vi "ReadAndPreprocessSensorValues.vi"(6 "Sensor References":T12, 8 "Force_calib_value":dbl, 9 "Velocity_calib_value":dbl, 10 "Control Loop Period [s]":dbl, 11 "Time [s]":dbl) -> (3 "RobotStateType":T13)   [LabVIEW 2019]
uses:
  ClusterType/RobotStateType.ctl
  <vilib>/myRIO/Instrument Drivers/Onboard IO/Encoder/typedefs/Encoder Reference.ctl
  <vilib>/myRIO/Common/Instrument Driver Framework/Utilities/typedefs/myRIO Generic Hardware Reference.ctl
  <vilib>/myRIO/Common/Instrument Driver Framework/Utilities/typedefs/Hardware Version Enum.ctl
  <vilib>/myRIO/Common/Instrument Driver Framework/Utilities/typedefs/myRIO v1.0 Reference.ctl
  <vilib>/myRIO/Common/Instrument Driver Framework/Utilities/typedefs/Generic FPGA Reference.ctl
  <vilib>/myRIO/Common/Instrument Driver Framework/myRIO v1.0/Encoder/typedefs/Encoder Channels Enum.ctl
  <vilib>/myRIO/Instrument Drivers/Onboard IO/AI/typedefs/AI Reference.ctl
  <vilib>/myRIO/Common/Instrument Driver Framework/myRIO v1.0/AI/typedefs/AI Channels List.ctl
  <vilib>/myRIO/Common/Instrument Driver Framework/myRIO v1.0/AI/typedefs/AI Channels Enum.ctl
  <vilib>/myRIO/Common/Instrument Driver Framework/Utilities/typedefs/Analog Scaling Constants List.ctl
  <vilib>/myRIO/Common/Instrument Driver Framework/Utilities/typedefs/Analog Scaling Constants.ctl
  <vilib>/Analysis/3filter.llb/Filter Passband Type.ctl
  <vilib>/Utility/error.llb/Error Cluster From Error Code.vi
  <vilib>/myRIO/Common/Instrument Driver Framework/myRIO v1.0/AI/vis/myRIO v1.0 Read AI.vi
  <vilib>/myRIO/Common/Instrument Driver Framework/myRIO v1.0/Encoder/vis/myRIO v1.0 Read Encoder.vi
  <vilib>/myRIO/Instrument Drivers/Onboard IO/Encoder/Encoder.lvlib
  <vilib>/myRIO/Instrument Drivers/Onboard IO/AI/AI.lvlib
  <vilib>/Analysis/NI_AALBase.lvlib
  <vilib>/ptbypt/NI_PtbyPt.lvlib
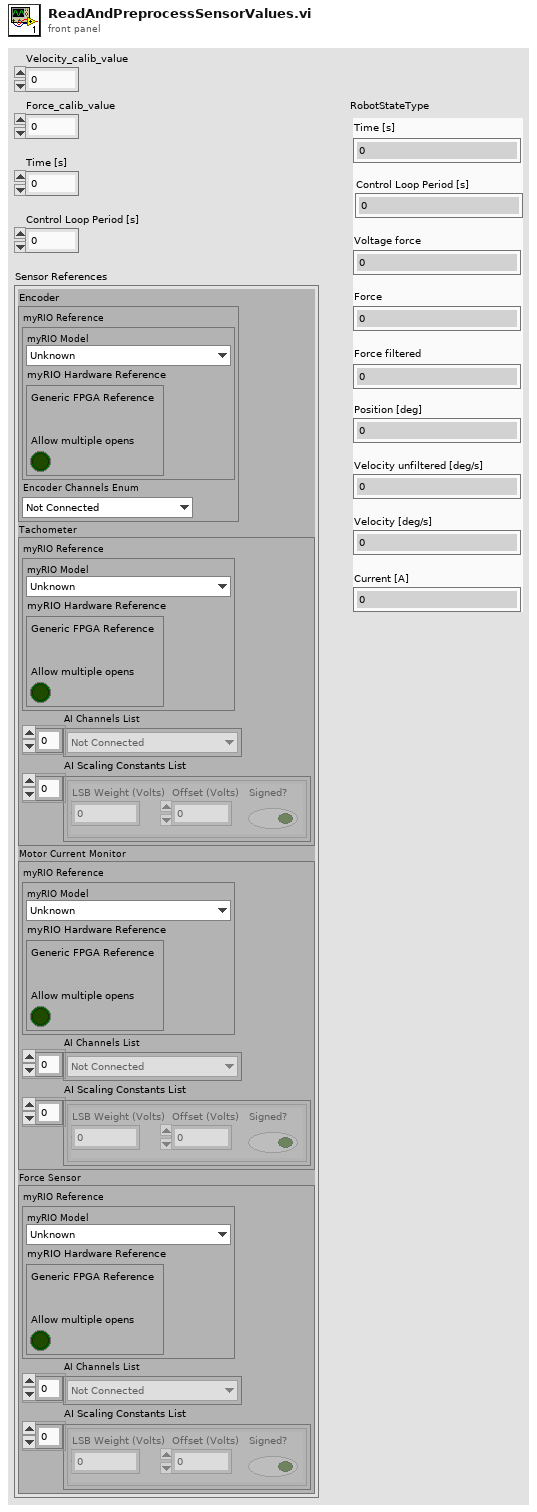
[diagram p1: front panel]
types:
  T1 = typedef "Encoder.lvlib/Encoder Reference.ctl" = cluster{"myRIO Reference":T2, "Encoder Channels Enum":T6}
  T2 = typedef "myRIO Generic Hardware Reference.ctl" = cluster{"myRIO Model":T3, "myRIO Hardware Reference":T4}
  T3 = typedef "Hardware Version Enum.ctl" = enum16{"Unknown", "myRIO-1900", "myRIO-1950", "roboRIO", "NI ELVIS RIO CM", "ELVIS III"}
  T4 = typedef "myRIO v1.0 Reference.ctl" = cluster{"Generic FPGA Reference":T5, "Allow multiple opens":bool}
  T5 = typedef "Generic FPGA Reference.ctl" = refnum<k20>
  T6 = typedef "Encoder Channels Enum.ctl" = enum16{"Not Connected", "C/ENC0", "C/ENC1", "A/ENC", "A/ENC0", "A/ENC1", "A/ENC2", "A/ENC3", "A/ENC4", "A/ENC5", "A/ENC6", "A/ENC7", "A/ENC8", "A/ENC9", "B/ENC", "B/ENC0", "B/ENC1", "B/ENC2", "B/ENC3", "B/ENC4", "B/ENC5", "B/ENC6", "B/ENC7", "B/ENC8", "B/ENC9", "DIO/ENC0", "DIO/ENC1", "DIO/ENC2", "DIO/ENC3", "DIO/ENC4"}
  T7 = typedef "AI.lvlib/AI Reference.ctl" = cluster{"myRIO Reference":T2, "AI Channels List":T8, "AI Scaling Constants List":T10}
  T8 = typedef "AI Channels List.ctl" = T9[]
  T9 = typedef "AI Channels Enum.ctl" = enum16{"Not Connected", "AudioIn/Left", "AudioIn/Right", "C/AI0", "C/AI1", "A/AI0", "A/AI1", "A/AI2", "A/AI3", "A/AI4", "A/AI5", "A/AI6", "A/AI7", "B/AI0", "B/AI1", "B/AI2", "B/AI3", "B/AI4", "B/AI5", "B/AI6", "B/AI7", "AI/AI0", "AI/AI1", "AI/AI2", "AI/AI3", "A/AI0 (DIFF)", "A/AI1 (DIFF)", "A/AI2 (DIFF)", "A/AI3 (DIFF)", "B/AI0 (DIFF)", "B/AI1 (DIFF)", "B/AI2 (DIFF)", "B/AI3 (DIFF)"}
  T10 = typedef "Analog Scaling Constants List.ctl" = T11[]
  T11 = typedef "Analog Scaling Constants.ctl" = cluster{"LSB Weight (Volts)":dbl, "Offset (Volts)":dbl, "Signed?":bool}
  T12 = cluster{"Encoder":T1, "Tachometer":T7, "Motor Current Monitor":T7, "Force Sensor":T7}
  T13 = typedef "RobotStateType.ctl" = cluster{"Time [s]":dbl, "Voltage force":dbl, "Force":dbl, "Force filtered":dbl, "Position [deg]":dbl, "Velocity unfiltered [deg/s]":dbl, "Velocity [deg/s]":dbl, "Current [A]":dbl, "Control Loop Period [s]":dbl}
  T14 = typedef "NI_AALBase.lvlib/Filter Passband Type.ctl" = enum32{"Lowpass", "Highpass", "Bandpass", "Bandstop"}
  T15 = typedef "TypeDefTachometerParam.ctl" = cluster{"Offset [V]":dbl, "Gain [deg/sV]":dbl}
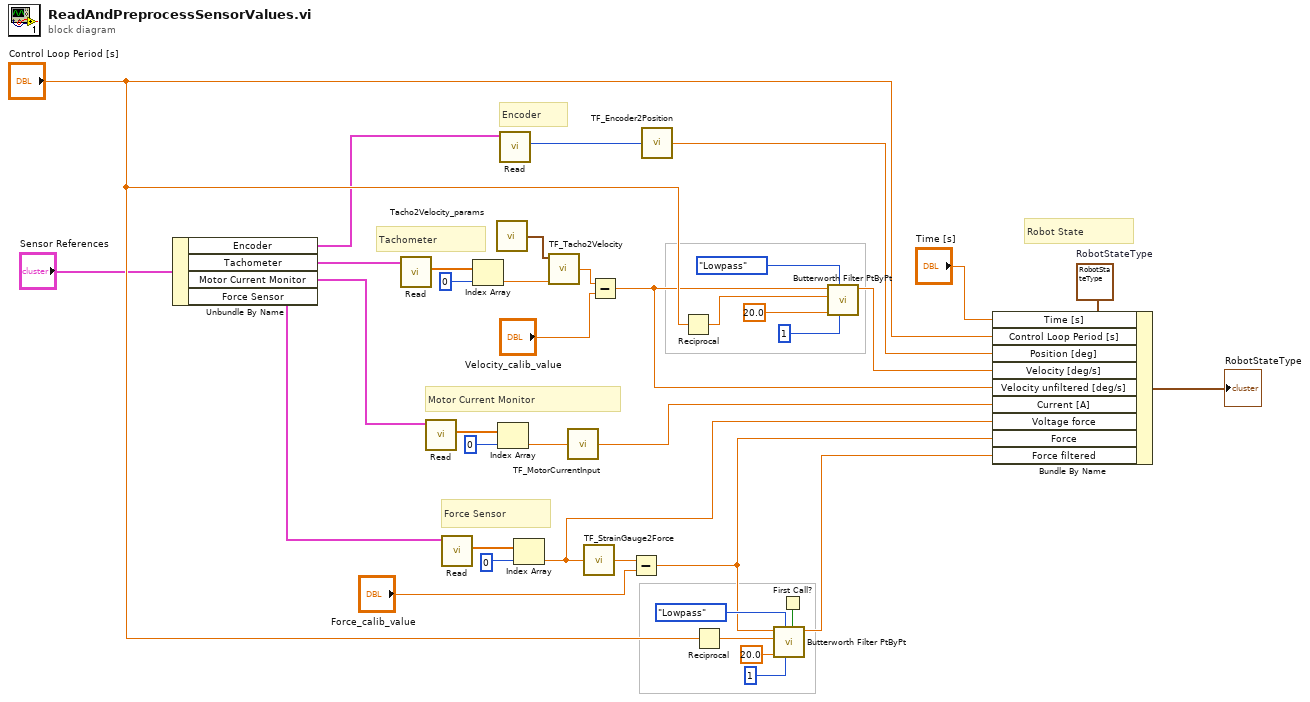
[diagram p0: block diagram]
diagram:
  w32 = T13 {"Time [s]"=0.0, "Voltage force"=0.0, "Force"=0.0, "Force filtered"=0.0, "Position [deg]"=0.0, "Velocity unfiltered [deg/s]"=0.0, "Velocity [deg/s]"=0.0, "Current [A]"=0.0, "Control Loop Period [s]"=0.0}  # RobotStateType
  # "Robot State"
  # "Force Sensor"
  # "Motor Current Monitor"
  # "Tachometer"
  # "Encoder"
  n1 = Unbundle By Name("Sensor References") -> ("Encoder"=w28:T1, "Tachometer"=w29:T7, "Motor Current Monitor"=w30:T7, "Force Sensor"=w31:T7)
  n2 = call <vilib>:"Read.vi"("AI Ref In"=w29) -> ("Values"=w10:dbl[])  [unwired: 8 in, 2 out]
  n3 = call <vilib>:"Read.vi"("AI Ref In"=w30) -> ("Values"=w11:dbl[])  [unwired: 8 in, 2 out]
  n4 = call <vilib>:"Read.vi"("AI Ref In"=w31) -> ("Values"=w15:dbl[])  [unwired: 8 in, 2 out]
  n5 = Index Array(array=w10, index=0) -> (element=w6:dbl)
  n6 = call "Tacho2Velocity_params.vi"() -> ("Cluster"=w5:T15)  [unwired: 5 in]
  n7 = Index Array(array=w11, index=0) -> (element=w13:dbl)
  n8 = call <vilib>:"Read.vi"("Encoder Ref In"=w28) -> ("Counter Value"=w8:i32)  [unwired: 6 in, 4 out]
  n9 = Index Array(array=w15, index=0) -> (element=w36:dbl)
  n10 = call "TF_Tacho2Velocity.vi"("Tachometer Voltage [V]"=w6, "Tachometer param"=w5) -> ("Tachometer Velocity [deg/s]"=w7:dbl)  [unwired: 2 in]
  n11 = call "TF_MotorCurrentInput.vi"("Motor Current Monitor Value [V]"=w13) -> ("Current [A]"=w33:dbl)
  n12 = call "TF_StrainGauge2Force.vi"("Strain Gauge Value [V]"=w36) -> ("Force [N]"=w25:dbl)  [unwired: 4 in]
  n13 = Subtract(x=w7, y="Velocity_calib_value") -> (x-y=w3:dbl)
  n14 = Subtract(x=w25, y="Force_calib_value") -> (x-y=w4:dbl)
  n15 = call "TF_Encoder2Position.vi"("Counter Value"=w8) -> ("Position [deg]"=w38:dbl)  [unwired: 4 in]
  n16 = Reciprocal(x="Control Loop Period [s]") -> (1/x=w17:dbl)
  n17 = Reciprocal(x="Control Loop Period [s]") -> (1/x=w21:dbl)
  n18 = First Call?() -> (First Call?: T/F=w16:bool)
  n19 = call <vilib>:"Butterworth Filter PtByPt.vi"("initialize"=w16, "order"=1, "filter type"=Filter_Passband_Type."Lowpass", "low cutoff freq: fl"=20.0, "sampling freq: fs"=w21, "x"=w4) -> ("Filtered x"=w1:dbl)  [unwired: 3 in, 1 out]
  n20 = call <vilib>:"Butterworth Filter PtByPt.vi"("order"=1, "filter type"=Filter_Passband_Type."Lowpass", "low cutoff freq: fl"=20.0, "sampling freq: fs"=w17, "x"=w3) -> ("Filtered x"=w2:dbl)  [unwired: 4 in, 1 out]
  n21 = Bundle By Name(cluster=w32, "Time [s]"="Time [s]", "Control Loop Period [s]"="Control Loop Period [s]", "Position [deg]"=w38, "Velocity [deg/s]"=w2, "Velocity unfiltered [deg/s]"=w3, "Current [A]"=w33, "Voltage force"=w36, "Force"=w4, "Force filtered"=w1) -> (→"RobotStateType":T13)
